vi "Read Name.vi"(11 "Build Package Item in":refnum<class "VIPM Item.lvclass">) -> (2 "Name":string)   [LabVIEW 2019, in "VIPM.lvlib" / "VIPM Item.lvclass"]
doc: "Returns the name of the solution item.\n----\nCopyright: MGI 2017\nAuthor: Derek Trepanier"
uses:
  VIPM Item.lvclass
  VIPM Item.lvclass/VIPM Item.ctl
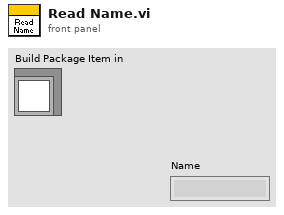
[diagram p1: front panel]
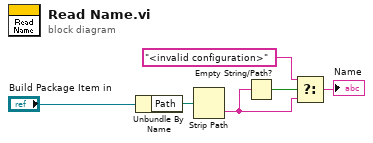
[diagram p0: block diagram]
diagram:
  n1 = Unbundle By Name("Build Package Item in") -> ("Path"=w5:path)
  n2 = Strip Path(path=w5) -> (name=w3:string)  [unwired: 1 out]
  n3 = Empty String/Path?(string/path=w3) -> (empty?=w4:bool)
  n4 = Select(t="<invalid configuration>", s=w4, f=w3) -> (s? t:f=→"Name":string)
